vi "DAQ Frequency Meter.vi"() -> ()   [LabVIEW 2013]
doc: "Use this template to build a standard state machine design pattern. Each state executes code and determines which state to transition to. Contrast this design pattern with the User Interface Event Handler pattern, in which code executes in response to user actions. Contrast this design pattern also with the Queued Message Handler pattern, in which each message handling code can queue zero or more new messages.\nNote: This template does not contain the most recent programming guidelines recommended by National Instruments. For a complete, project-based implementation of the Standard State Machine pattern, use the Create Project dialog box instead of this template."
uses:
  DAQ_Count_States.ctl
  <vilib>/DAQmx/read.llb/DAQmx Read (Counter DBL 1Chan 1Samp).vi
  <vilib>/DAQmx/create/channels.llb/DAQmx Create Channel (CI-Frequency).vi
  <vilib>/DAQmx/create/channels.llb/DAQmx Create Channel (CI-Period).vi
  <vilib>/DAQmx/miscellaneous.llb/DAQmx Fill In Error Info.vi
  <resource>/objmgr/daqmx.rc
panel:
  in  "stop":bool
  out "data":dbl caption="Frequency, Hz" format="%_8g"
  in  "mode":enum16{"period", "frequency"}(ring)
  in  "terminal":tag
  in  "counter":tag
  in  "minimum value":dbl=2.0 format="%0.6f"
  in  "maximum value":dbl=100.0 format="%0.6f"
  in  "measurement method":i32(ring)=10105 items=["Low Frequency with 1 Counter"=10105, "High Frequency with 2 Counters"=10157, "Large Range with 2 Counters"=10205, "Dynamic Averaging"=16065]
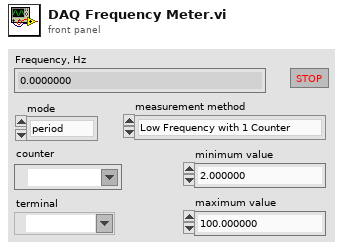
[diagram p1: front panel]
types:
  T1 = typedef "DAQ_Count_States.ctl" = enum16{"Initialize", "Read", "Stop"}
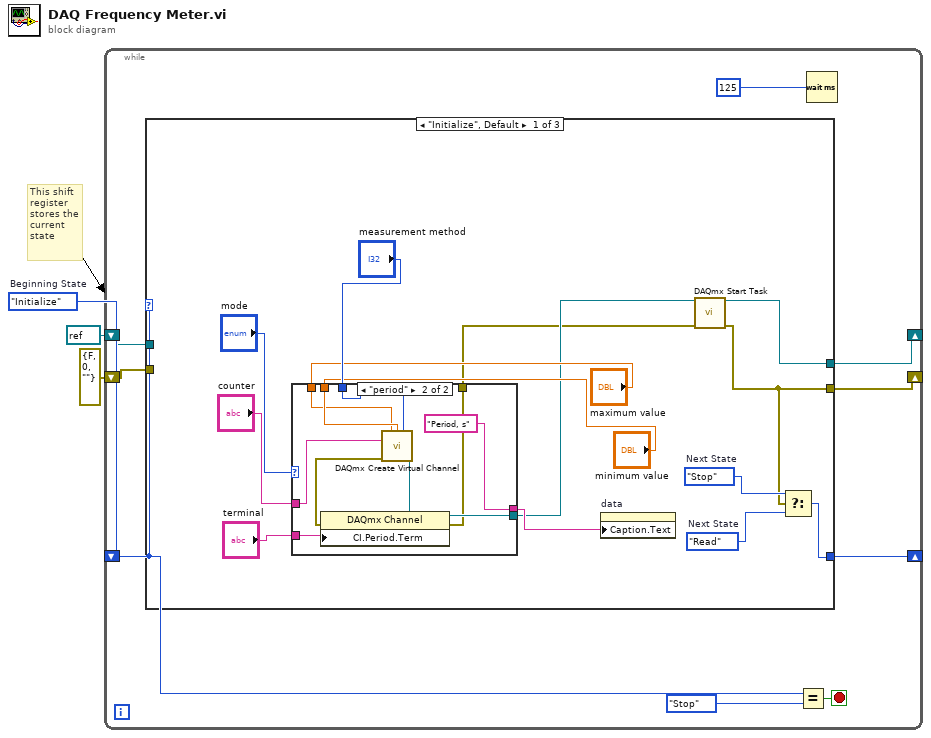
[diagram p0: block diagram]
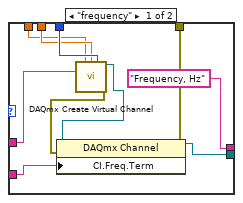
[diagram p2: hidden frame]
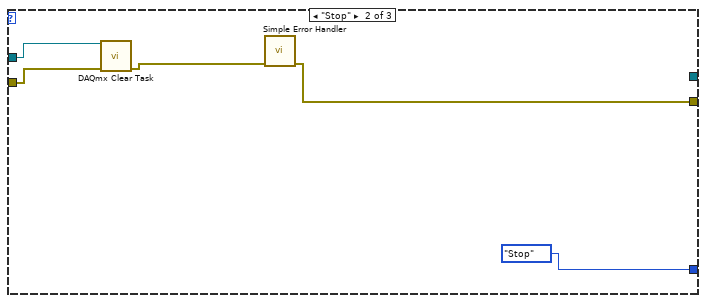
[diagram p3: hidden frame]
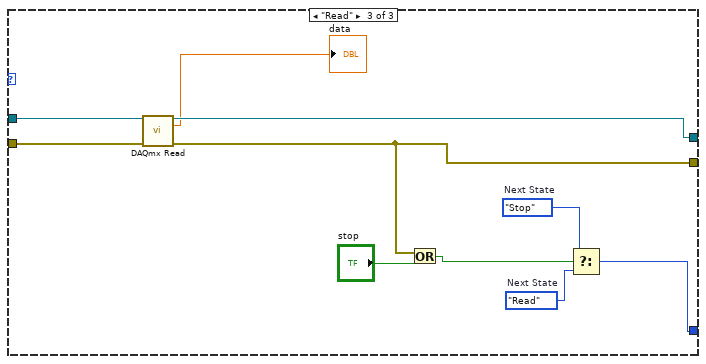
[diagram p4: hidden frame]
diagram:
  w3 = DAQ_Count_States."Initialize"  # Beginning State
  # "This shift\nregister\nstores the\ncurrent\nstate"
  n1 = while {
    shift-right: [w9] -> _
    shift-left: w3 -> [w10]
    shift-right: [w7] -> _
    shift-left: refnum<k21> refnum ("task out") -> [w5]
    shift-right: [w6] -> _
    shift-left: errorcluster {"status"=FALSE, "code"=0, "source"=""} ("error out") -> [w4]
    stop <- w12 stop-if-true
    n2 = case shown="\"Initialize\", Default" w10 {
      tunnel: [w18 DAQ_Count_States."Stop" ("Next State") w52] -> w9
      tunnel: [w26 _ w59] -> w7
      tunnel: [w15 w47 w56] -> w6
      tunnel: w5 -> [_ w50 w61]
      tunnel: w4 -> [_ w49 w60]
      frame "Initialize", Default {
        w17 = DAQ_Count_States."Stop"  # Next State
        w16 = DAQ_Count_States."Read"  # Next State
        n3 = case shown="\"period\"" "mode" {
          tunnel: "terminal" -> [w36 w46]
          tunnel: "measurement method" -> [w35 w45]
          tunnel: "minimum value" -> [w34 w44]
          tunnel: "maximum value" -> [w31 w43]
          tunnel: "counter" -> [w33 w42]
          tunnel: ["Frequency, Hz" "Period, s"] -> w19
          tunnel: [w30 w38] -> w14
          tunnel: [w29 w37] -> w13
          frame "frequency" {
            n4 = call-poly <vilib>:"DAQmx Create Virtual Channel.vi"("maximum value"=w31, "minimum value"=w34, "measurement method"=w35, "counter"=w33) -> ("task out"=w27:refnum<k21>, "error out"=w28:errorcluster)  [unwired: 10 in]
            n5 = property class="DAQmx Channel"(reference=w27, error in=w28, "CI.Freq.Term"=w36) -> (reference out=w30:refnum<k21>, error out=w29:errorcluster)
          }
          frame "period" {
            n6 = call-poly <vilib>:"DAQmx Create Virtual Channel.vi"("maximum value"=w43, "minimum value"=w44, "measurement method"=w45, "counter"=w42) -> ("task out"=w40:refnum<k21>, "error out"=w39:errorcluster)  [unwired: 10 in]
            n7 = property class="DAQmx Channel"(reference=w40, error in=w39, "CI.Period.Term"=w46) -> (reference out=w38:refnum<k21>, error out=w37:errorcluster)
          }
        }
        n8 = property on="data" class="DigNum (strict)"("Caption.Text"=w19) -> ()  [unwired: 2 in, 2 out]
        n9 = call <vilib>:"DAQmx Start Task.vi"("task/channels in"=w14, "error in"=w13) -> ("task out"=w26:refnum<k21>, "error out"=w15:errorcluster)  [unwired: 12 in]
        n10 = Select(t=w17, s=w15, f=w16) -> (s? t:f=w18:T1)
      }
      frame "Stop" {
        n11 = call <vilib>:"DAQmx Clear Task.vi"("task in"=w50, "error in"=w49) -> ("error out"=w48:errorcluster)  [unwired: 13 in]
        n12 = call <vilib>:"Simple Error Handler.vi"("error in (no error)"=w48) -> ("error out"=w47:errorcluster)  [unwired: 4 in, 4 out]
      }
      frame "Read" {
        w53 = DAQ_Count_States."Read"  # Next State
        w54 = DAQ_Count_States."Stop"  # Next State
        n13 = call-poly <vilib>:"DAQmx Read.vi"("task/channels in"=w61, "error in"=w60) -> ("task out"=w59:refnum<k21>, "data"=→"data":dbl, "error out"=w56:errorcluster)  [unwired: 11 in]
        n14 = Or(x=w56, y="stop") -> (x .or. y?=w55:bool)
        n15 = Select(t=w54, s=w55, f=w53) -> (s? t:f=w52:T1)
      }
    }
    n16 = Equal?(x=w10, y=DAQ_Count_States."Stop" ("States")) -> (x = y?=w12:bool)
    n17 = Wait (ms)(milliseconds to wait=u32 125) -> ()  [unwired: 1 out]
  }
